vi "Master3.vi"   [LabVIEW 2016, in "Moving Motor.lvrbt"]
uses:
  Moving Motor.lvrbt
  <vilib>/NXT/Block Support/NXT_InputPort.ctl
  <vilib>/NXT/Hardware/Plugins/Tetrix DC Motor/TetrixDCMotorAddress.ctl
  <vilib>/NXT/Hardware/Plugins/Tetrix 180 deg Servo/Tetrix180ServoAddress.ctl
  <vilib>/NXT/Dual Mode Library/Sensors/EV3_Color_Color.vi
  <vilib>/NXT/NXTIO Xnodes/NXTIONodeSubVIs/TETRIX IO Move Servos.vi
  <vilib>/NXT/NXTIO Xnodes/NXTIONodeSubVIs/TETRIX IO Move DC Motors.vi
  <vilib>/NXT/NXTIO Xnodes/NXTIONodeSubVIs/TETRIX IO Stop DC Motors.vi
  <vilib>/NXT/NXTIO Xnodes/AddressXNode/NXTIOAddress.xnode
  <vilib>/NXT/NXTIO Xnodes/NXTIOXNode/NXTIO.xnode
  <vilib>/NXT/Subs/LVHSConnector.ctl
  <vilib>/NXT/LegoClasses/BrickReference/BrickReference.lvclass
types:
  T1 = typedef "NXT_InputPort.ctl" = u32
  T2 = typedef "LVHSConnector.ctl" = refnum<class "BrickReference.lvclass">
  T3 = typedef "Tetrix180ServoAddress.ctl" = i32
  T4 = cluster{"Tetrix180Servo":T3, "Tetrix180Servo":T3}
  T5 = typedef "TetrixDCMotorAddress.ctl" = i32
  T6 = cluster{"TetrixDCMotor":T5, "TetrixDCMotor 2":T5}
  T7 = typedef "ColorSensorColors.ctl" = enum16{"No Color", "Black", "Blue", "Green", "Yellow", "Red", "White", "Brown"}
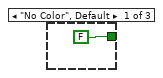
[diagram p2: hidden frame]
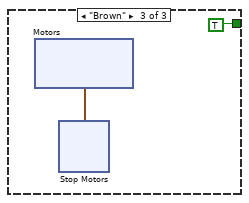
[diagram p3: hidden frame]
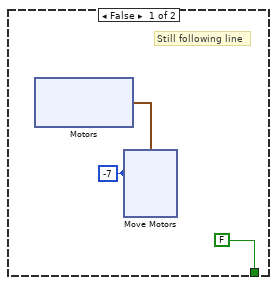
[diagram p4: hidden frame]
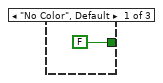
[diagram p5: hidden frame]
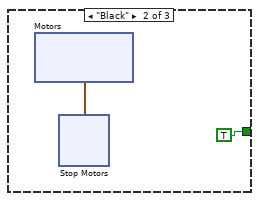
[diagram p6: hidden frame]
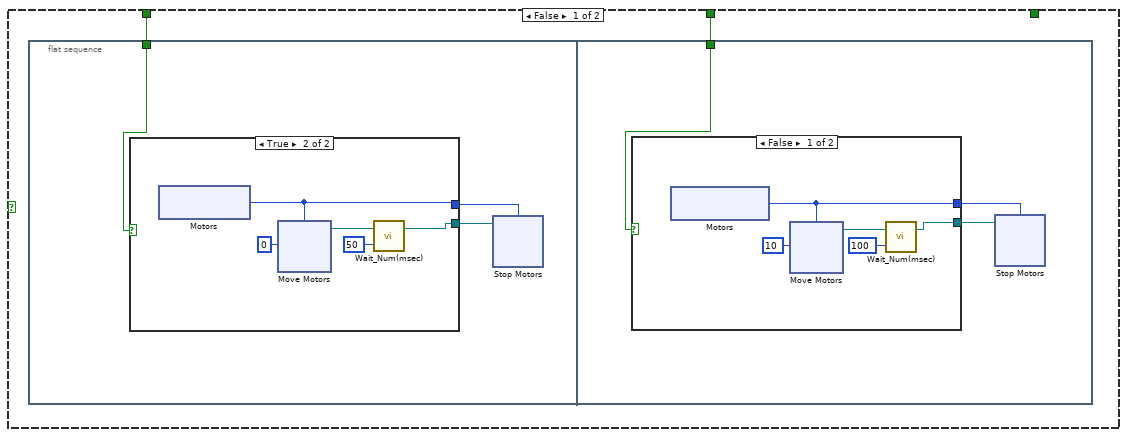
[diagram p7: hidden frame]
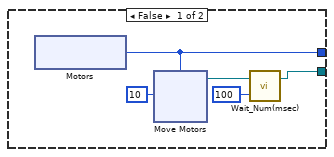
[diagram p8: hidden frame]
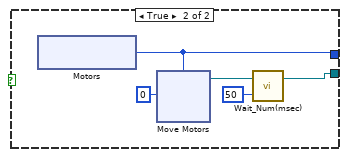
[diagram p9: hidden frame]
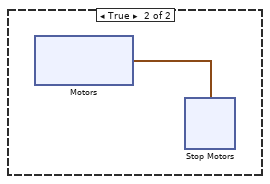
[diagram p10: hidden frame]
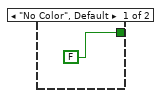
[diagram p11: hidden frame]
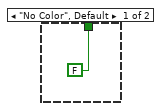
[diagram p12: hidden frame]
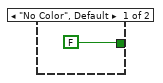
[diagram p13: hidden frame]
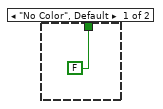
[diagram p14: hidden frame]
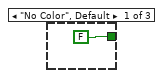
[diagram p15: hidden frame]
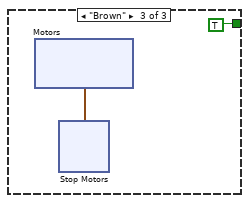
[diagram p16: hidden frame]
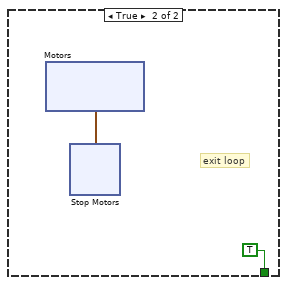
[diagram p17: hidden frame]
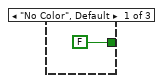
[diagram p18: hidden frame]
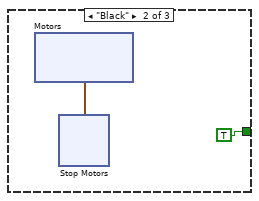
[diagram p19: hidden frame]
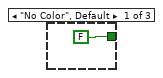
[diagram p20: hidden frame]
diagram:
  w2 = i8 8 ("Power/Speed 1")
  w12 = i8 -16 ("Power/Speed 1")
  w31 = i8 10 ("Power/Speed 1")
  w33 = i8 0 ("Power/Speed 1")
  w45 = i8 -8 ("Power/Speed 1")
  w50 = T1 5 items=["Port 1"=0, "Port 2"=1, "Port 3"=2, "Port 4"=3, "MidRightColor"=5] ("Port (Port 1)")
  w51 = T1 6 items=["Port 1"=0, "Port 2"=1, "Port 3"=2, "Port 4"=3, "MidLeftColor"=6] ("Port (Port 1)")
  w52 = T1 4 items=["Port 1", "Port 2", "Port 3", "Port 4", "RightColor"] ("Port (Port 1)")
  w53 = T1 7 items=["Port 1"=0, "Port 2"=1, "Port 3"=2, "Port 4"=3, "LeftColor"=7] ("Port (Port 1)")
  w70 = i8 -8 ("Power/Speed 1")
  w81 = i8 10 ("Power/Speed 1")
  w80 = i8 0 ("Power/Speed 1")
  # "arm lifting"
  # "Go forward"
  # "Initialize"
  # "Go to intersection"
  # "Turn right"
  # "Combination of line follower and dual-edge detector"
  # "Move backward and turn right to enter the line"
  # "Stop this motor instance"
  # "Stop when it detects the first fat tape"
  # "Let it run for 1s to pass that first thin tape"
  # "Initialize"
  n1 = call-poly <vilib>:"PolySensor.vi"("Port (Port 1)"=w52) -> ("NXT/EV3"=w49:T2)  [unwired: 2 in, 1 out]
  n2 = call-poly <vilib>:"PolySensor.vi"("NXT/EV3"=w49, "Port (Port 1)"=w50) -> ("NXT/EV3"=w48:T2)  [unwired: 1 in, 1 out]
  n3 = call-poly <vilib>:"PolySensor.vi"("NXT/EV3"=w48, "Port (Port 1)"=w51) -> ("NXT/EV3"=w47:T2)  [unwired: 1 in, 1 out]
  n4 = call-poly <vilib>:"PolySensor.vi"("NXT/EV3"=w47, "Port (Port 1)"=w53) -> ("NXT/EV3"=w46:T2)  [unwired: 1 in, 1 out]
  n5 = xnode "Motors"() -> ("Motor"=w78:T4)
  n6 = xnode "Move Servos"("Position 2"=u8 0, "Position 1"=u8 0, "Motors"=w78, "NXT/EV3"=w46) -> ("NXT/EV3"=w79:T2)
  n7 = xnode "Motors"() -> ("Motor"=w58:cluster{"TetrixDCMotor":T5, "TetrixDCMotor":T5})
  n8 = xnode "Move Motors"("Power/Speed 2"=w80, "Power/Speed 1"=w80, "Motors"=w58, "NXT/EV3"=w79) -> ("NXT/EV3"=w86:T2)
  n9 = call <vilib>:"Wait_Num(msec).vi"("Time (100 msec)"=u32 100, "NXT/EV3"=w86) -> ("NXT/EV3"=w82:T2)  [unwired: 2 in]
  n10 = xnode "Move Motors"("Power/Speed 2"=w81, "Power/Speed 1"=w81, "Motors"=w58, "NXT/EV3"=w82) -> ("NXT/EV3"=w84:T2)
  n11 = call <vilib>:"Wait_Num(msec).vi"("Time (100 msec)"=u32 1200, "NXT/EV3"=w84) -> ("NXT/EV3"=w59:T2)  [unwired: 2 in]
  n12 = xnode "Stop Motors"("Motors"=w58, "NXT/EV3"=w59) -> ("NXT/EV3"=w56:T2)
  n13 = call <vilib>:"Wait_Num(msec).vi"("Time (100 msec)"=u32 500, "NXT/EV3"=w56) -> ("NXT/EV3"=w55:T2)  [unwired: 2 in]
  n14 = while {
    tunnel: [w90] -> w72
    tunnel: w55 -> [w87]
    stop <- w91 stop-if-true
    w94 = T1 4 items=["Port 1", "Port 2", "Port 3", "Port 4", "RightColor"] ("Port (Port 1)")
    w96 = T1 7 items=["Port 1"=0, "Port 2"=1, "Port 3"=2, "Port 4"=3, "LeftColor"=7] ("Port (Port 1)")
    n15 = call-poly <vilib>:"PolySensor.vi"("Port (Port 1)"=w96) -> ("Detected Color"=w95:T7)  [unwired: 2 in, 1 out]
    n16 = call-poly <vilib>:"PolySensor.vi"("Port (Port 1)"=w94) -> ("Detected Color"=w93:T7)  [unwired: 2 in, 1 out]
    n17 = case shown="\"Black\"" w95 {
      tunnel: [FALSE TRUE TRUE] -> w89
      tunnel: w87 -> [_ w139 _]
      tunnel: w87 -> [_ _ w148]
      frame "No Color", Default {
      }
      frame "Black" {
        n18 = xnode "Motors"() -> ("Motor"=w141:cluster{"TetrixDCMotor":T5, "TetrixDCMotor":T5})
        n19 = xnode "Stop Motors"("Motors"=w141, "NXT/EV3"=w139) -> ()  [unwired: 1 out]
      }
      frame "Brown" {
        n20 = xnode "Motors"() -> ("Motor"=w149:cluster{"TetrixDCMotor":T5, "TetrixDCMotor":T5})
        n21 = xnode "Stop Motors"("Motors"=w149, "NXT/EV3"=w148) -> ()  [unwired: 1 out]
      }
    }
    n22 = case shown="\"Black\"" w93 {
      tunnel: [FALSE TRUE TRUE] -> w88
      tunnel: w87 -> [_ w98 w107]
      frame "No Color", Default {
      }
      frame "Black" {
        n23 = xnode "Motors"() -> ("Motor"=w99:cluster{"TetrixDCMotor":T5, "TetrixDCMotor":T5})
        n24 = xnode "Stop Motors"("Motors"=w99, "NXT/EV3"=w98) -> ()  [unwired: 1 out]
      }
      frame "Brown" {
        n25 = xnode "Motors"() -> ("Motor"=w108:cluster{"TetrixDCMotor":T5, "TetrixDCMotor":T5})
        n26 = xnode "Stop Motors"("Motors"=w108, "NXT/EV3"=w107) -> ()  [unwired: 1 out]
      }
    }
    n27 = Or(x=w89, y=w88) -> (x .or. y?=w92:bool)
    n28 = case shown="False" w92 {
      tunnel: [FALSE TRUE] -> w91
      tunnel: [w116 w129] -> w90
      frame False {
        w119 = i8 5 ("Power/Speed 1")
        n29 = xnode "Motors"() -> ("Motor"=w118:cluster{"TetrixDCMotor":T5, "TetrixDCMotor":T5})
        n30 = xnode "Move Motors"("Power/Speed 2"=w119, "Power/Speed 1"=w119, "Motors"=w118) -> ("NXT/EV3"=w116:T2)  [unwired: 1 in]
      }
      frame True {
        n31 = xnode "Motors"() -> ("Motor"=w130:cluster{"TetrixDCMotor":T5, "TetrixDCMotor":T5})
        n32 = xnode "Stop Motors"("Motors"=w130) -> ("NXT/EV3"=w129:T2)  [unwired: 1 in]
      }
    }
  }
  n33 = call <vilib>:"Wait_Num(msec).vi"("Time (100 msec)"=u32 1000, "NXT/EV3"=w72) -> ("NXT/EV3"=w71:T2)  [unwired: 2 in]
  n34 = xnode "Motors"() -> ("Motor"=w63:cluster{"TetrixDCMotor":T5, "TetrixDCMotor":T5})
  n35 = xnode "Move Motors"("Power/Speed 2"=w70, "Power/Speed 1"=w70, "Motors"=w63, "NXT/EV3"=w71) -> ("NXT/EV3"=w68:T2)
  n36 = call <vilib>:"Wait_Num(msec).vi"("Time (100 msec)"=u32 700, "NXT/EV3"=w68) -> ("NXT/EV3"=w64:T2)  [unwired: 2 in]
  n37 = xnode "Stop Motors"("Motors"=w63, "NXT/EV3"=w64) -> ("NXT/EV3"=w62:T2)
  n38 = xnode "Move Motors"("Power/Speed 2"=i8 0, "Power/Speed 1"=i8 16, "Motors"=w63, "NXT/EV3"=w62) -> ("NXT/EV3"=w65:T2)
  n39 = call <vilib>:"Wait_Num(msec).vi"("Time (100 msec)"=u32 1800, "NXT/EV3"=w65) -> ("NXT/EV3"=w74:T2)  [unwired: 2 in]
  n40 = xnode "Stop Motors"("Motors"=w63, "NXT/EV3"=w74) -> ("NXT/EV3"=w60:T2)
  n41 = call <vilib>:"Wait_Num(msec).vi"("Time (100 msec)"=u32 1000, "NXT/EV3"=w60) -> ("NXT/EV3"=w54:T2)  [unwired: 2 in]
  n42 = while {
    tunnel: [w157] -> w43
    tunnel: w54 -> [_]
    stop <- w160 stop-if-true
    w163 = T1 7 items=["Port 1"=0, "Port 2"=1, "Port 3"=2, "Port 4"=3, "LeftColor"=4, "RightColor"=7] ("Port (Port 1)")
    w165 = T1 4 items=["Port 1"=0, "Port 2"=1, "Port 3"=2, "Port 4"=3, "LeftColor"=4, "RightColor"=7] ("Port (Port 1)")
    n43 = call-poly <vilib>:"PolySensor.vi"("Port (Port 1)"=w165) -> ("Detected Color"=w164:T7)  [unwired: 2 in, 1 out]
    n44 = call-poly <vilib>:"PolySensor.vi"("Port (Port 1)"=w163) -> ("Detected Color"=w162:T7, "NXT/EV3"=w157:T2)  [unwired: 2 in]
    n45 = case shown="\"Brown\"" w164 {
      tunnel: [FALSE TRUE TRUE] -> w159
      frame "No Color", Default {
      }
      frame "Black" {
        n46 = xnode "Motors"() -> ("Motor"=w205:cluster{"TetrixDCMotor":T5, "TetrixDCMotor":T5})
        n47 = xnode "Stop Motors"("Motors"=w205) -> ()  [unwired: 1 in, 1 out]
      }
      frame "Brown" {
        n48 = xnode "Motors"() -> ("Motor"=w212:cluster{"TetrixDCMotor":T5, "TetrixDCMotor":T5})
        n49 = xnode "Stop Motors"("Motors"=w212) -> ()  [unwired: 1 in, 1 out]
      }
    }
    n50 = case shown="\"Black\"" w162 {
      tunnel: [FALSE TRUE TRUE] -> w158
      frame "No Color", Default {
      }
      frame "Black" {
        n51 = xnode "Motors"() -> ("Motor"=w167:cluster{"TetrixDCMotor":T5, "TetrixDCMotor":T5})
        n52 = xnode "Stop Motors"("Motors"=w167) -> ()  [unwired: 1 in, 1 out]
      }
      frame "Brown" {
        n53 = xnode "Motors"() -> ("Motor"=w175:cluster{"TetrixDCMotor":T5, "TetrixDCMotor":T5})
        n54 = xnode "Stop Motors"("Motors"=w175) -> ()  [unwired: 1 in, 1 out]
      }
    }
    n55 = Or(x=w159, y=w158) -> (x .or. y?=w161:bool)
    n56 = case shown="False" w161 {
      tunnel: [FALSE TRUE] -> w160
      frame False {
        w184 = i8 7 ("Power/Speed 1")
        # "Still following line"
        n57 = xnode "Motors"() -> ("Motor"=w183:cluster{"TetrixDCMotor":T5, "TetrixDCMotor":T5})
        n58 = xnode "Move Motors"("Power/Speed 2"=w184, "Power/Speed 1"=w184, "Motors"=w183) -> ()  [unwired: 1 in, 1 out]
      }
      frame True {
        # "exit loop"
        n59 = xnode "Motors"() -> ("Motor"=w195:cluster{"TetrixDCMotor":T5, "TetrixDCMotor":T5})
        n60 = xnode "Stop Motors"("Motors"=w195) -> ()  [unwired: 1 in, 1 out]
      }
    }
  }
  n61 = call <vilib>:"Wait_Num(msec).vi"("Time (100 msec)"=u32 200, "NXT/EV3"=w43) -> ("NXT/EV3"=w42:T2)  [unwired: 2 in]
  n62 = xnode "Motors"() -> ("Motor"=w44:cluster{"TetrixDCMotor":T5, "TetrixDCMotor":T5})
  n63 = xnode "Move Motors"("Power/Speed 2"=w45, "Power/Speed 1"=w45, "Motors"=w44, "NXT/EV3"=w42) -> ("NXT/EV3"=w39:T2)
  n64 = call <vilib>:"Wait_Num(msec).vi"("Time (100 msec)"=u32 500, "NXT/EV3"=w39) -> ("NXT/EV3"=w38:T2)  [unwired: 2 in]
  n65 = while {
    tunnel: w38 -> [_]
    tunnel: [w220] -> w36
    stop <- w221 stop-if-true
    w232 = T1 5 items=["Port 1"=0, "Port 2"=1, "Port 3"=2, "Port 4"=3, "MidRightColor"=5] ("Port (Port 1)")
    w233 = T1 6 items=["Port 1"=0, "Port 2"=1, "Port 3"=2, "Port 4"=3, "MidLeftColor"=6] ("Port (Port 1)")
    w234 = T1 4 items=["Port 1", "Port 2", "Port 3", "Port 4", "RightColor"] ("Port (Port 1)")
    w235 = T1 7 items=["Port 1"=0, "Port 2"=1, "Port 3"=2, "Port 4"=3, "LeftColor"=7] ("Port (Port 1)")
    n66 = call-poly <vilib>:"PolySensor.vi"("Port (Port 1)"=w234) -> ("Detected Color"=w228:T7, "NXT/EV3"=w220:T2)  [unwired: 2 in]
    n67 = call-poly <vilib>:"PolySensor.vi"("Port (Port 1)"=w235) -> ("Detected Color"=w231:T7)  [unwired: 2 in, 1 out]
    n68 = call-poly <vilib>:"PolySensor.vi"("Port (Port 1)"=w233) -> ("Detected Color"=w230:T7)  [unwired: 2 in, 1 out]
    n69 = call-poly <vilib>:"PolySensor.vi"("Port (Port 1)"=w232) -> ("Detected Color"=w229:T7)  [unwired: 2 in, 1 out]
    n70 = case shown="\"Black\"" w231 {
      tunnel: [FALSE TRUE] -> w224
      frame "No Color", Default {
      }
      frame "Black" {
      }
    }
    n71 = case shown="\"Black\"" w230 {
      tunnel: [FALSE TRUE] -> w227
      frame "No Color", Default {
      }
      frame "Black" {
      }
    }
    n72 = case shown="\"Black\"" w229 {
      tunnel: [FALSE TRUE] -> w226
      frame "No Color", Default {
      }
      frame "Black" {
      }
    }
    n73 = case shown="\"Black\"" w228 {
      tunnel: [FALSE TRUE] -> w223
      frame "No Color", Default {
      }
      frame "Black" {
      }
    }
    n74 = And "LC & RC"(x=w224, y=w223) -> (x .and. y?=w225:bool)
    n75 = And "MLC & MRC"(x=w227, y=w226) -> (x .and. y?=w222:bool)
    n76 = case shown="True" w225 {
      tunnel: w224 -> [w237 _]
      tunnel: w223 -> [w236 _]
      tunnel: w222 -> [_ w306]
      frame False {
        n77 = flat-sequence {
          tunnel: w237 -> [w238]
          tunnel: w236 -> [w272]
          frame #0 {
            n78 = case shown="True" w238 {
              tunnel: [w247 w259] -> w240
              tunnel: [w246 w260] -> w239
              frame False {
                n79 = xnode "Motors"() -> ("Motor"=w246:T5)
                n80 = xnode "Move Motors"("Power/Speed 1"=i8 10, "Motors"=w246) -> ("NXT/EV3"=w249:T2)  [unwired: 1 in]
                n81 = call <vilib>:"Wait_Num(msec).vi"("Time (100 msec)"=u32 100, "NXT/EV3"=w249) -> ("NXT/EV3"=w247:T2)  [unwired: 2 in]
              }
              frame True {
                n82 = xnode "Motors"() -> ("Motor"=w260:T5)
                n83 = xnode "Move Motors"("Power/Speed 1"=i8 0, "Motors"=w260) -> ("NXT/EV3"=w262:T2)  [unwired: 1 in]
                n84 = call <vilib>:"Wait_Num(msec).vi"("Time (100 msec)"=u32 50, "NXT/EV3"=w262) -> ("NXT/EV3"=w259:T2)  [unwired: 2 in]
              }
            }
            n85 = xnode "Stop Motors"("Motors"=w239, "NXT/EV3"=w240) -> ()  [unwired: 1 out]
          }
          frame #1 {
            n86 = case shown="False" w272 {
              tunnel: [w281 w293] -> w274
              tunnel: [w280 w294] -> w273
              frame False {
                n87 = xnode "Motors"() -> ("Motor"=w280:T5)
                n88 = xnode "Move Motors"("Power/Speed 1"=i8 10, "Motors"=w280) -> ("NXT/EV3"=w283:T2)  [unwired: 1 in]
                n89 = call <vilib>:"Wait_Num(msec).vi"("Time (100 msec)"=u32 100, "NXT/EV3"=w283) -> ("NXT/EV3"=w281:T2)  [unwired: 2 in]
              }
              frame True {
                n90 = xnode "Motors"() -> ("Motor"=w294:T5)
                n91 = xnode "Move Motors"("Power/Speed 1"=i8 0, "Motors"=w294) -> ("NXT/EV3"=w296:T2)  [unwired: 1 in]
                n92 = call <vilib>:"Wait_Num(msec).vi"("Time (100 msec)"=u32 50, "NXT/EV3"=w296) -> ("NXT/EV3"=w293:T2)  [unwired: 2 in]
              }
            }
            n93 = xnode "Stop Motors"("Motors"=w273, "NXT/EV3"=w274) -> ()  [unwired: 1 out]
          }
        }
      }
      frame True {
        n94 = case shown="False" w306 {
          frame False {
            n95 = xnode "Motors"() -> ("Motor"=w312:cluster{"TetrixDCMotor":T5, "TetrixDCMotor":T5})
            n96 = xnode "Stop Motors"("Motors"=w312) -> ("NXT/EV3"=w318:T2)  [unwired: 1 in]
            n97 = call <vilib>:"Wait_Num(msec).vi"("Time (100 msec)"=u32 50, "NXT/EV3"=w318) -> ("NXT/EV3"=w313:T2)  [unwired: 2 in]
            n98 = xnode "Move Motors"("Power/Speed 2"=i8 0, "Power/Speed 1"=i8 -9, "Motors"=w312, "NXT/EV3"=w313) -> ("NXT/EV3"=w315:T2)
            n99 = call <vilib>:"Wait_Num(msec).vi"("Time (100 msec)"=u32 800, "NXT/EV3"=w315) -> ("NXT/EV3"=w319:T2)  [unwired: 2 in]
            n100 = xnode "Stop Motors"("Motors"=w312, "NXT/EV3"=w319) -> ("NXT/EV3"=w309:T2)
            n101 = xnode "Move Motors"("Power/Speed 2"=i8 -9, "Power/Speed 1"=i8 0, "Motors"=w312, "NXT/EV3"=w309) -> ("NXT/EV3"=w307:T2)
            n102 = call <vilib>:"Wait_Num(msec).vi"("Time (100 msec)"=u32 800, "NXT/EV3"=w307) -> ()  [unwired: 2 in, 1 out]
          }
          frame True {
            n103 = xnode "Motors"() -> ("Motor"=w348:cluster{"TetrixDCMotor":T5, "TetrixDCMotor":T5})
            n104 = xnode "Stop Motors"("Motors"=w348) -> ()  [unwired: 1 in, 1 out]
          }
        }
      }
    }
    n105 = And "Only exit loop when all 4 sensors detect black"(x=w225, y=w222) -> (x .and. y?=w221:bool)
  }
  n106 = xnode "Motors"() -> ("Motor"=w17:T4)
  n107 = call <vilib>:"Wait_Num(msec).vi"("Time (100 msec)"=u32 200, "NXT/EV3"=w36) -> ("NXT/EV3"=w19:T2)  [unwired: 2 in]
  n108 = xnode "Move Servos"("Position 2"=u8 54, "Position 1"=u8 0, "Motors"=w17, "NXT/EV3"=w19) -> ("NXT/EV3"=w32:T2)
  n109 = xnode "Motors"() -> ("Motor"=w24:cluster{"TetrixDCMotor":T5, "TetrixDCMotor":T5})
  n110 = xnode "Move Motors"("Power/Speed 2"=w33, "Power/Speed 1"=w33, "Motors"=w24, "NXT/EV3"=w32) -> ("NXT/EV3"=w28:T2)
  n111 = xnode "Move Motors"("Power/Speed 2"=w31, "Power/Speed 1"=w31, "Motors"=w24, "NXT/EV3"=w28) -> ("NXT/EV3"=w29:T2)
  n112 = call-poly <vilib>:"PolyWait.vi"("Time (100 msec)"=u32 1000, "NXT/EV3"=w29) -> ("NXT/EV3"=w27:T2)  [unwired: 2 in]
  n113 = xnode "Stop Motors"("Motors"=w24, "NXT/EV3"=w27) -> ("NXT/EV3"=w22:T2)
  n114 = xnode "Move Servos"("Position 2"=u8 0, "Position 1"=u8 0, "Motors"=w17, "NXT/EV3"=w22) -> ("NXT/EV3"=w20:T2)
  n115 = call-poly <vilib>:"PolyWait.vi"("Time (100 msec)"=u32 2000, "NXT/EV3"=w20) -> ("NXT/EV3"=w15:T2)  [unwired: 2 in]
  n116 = xnode "Move Servos"("Position 2"=u8 120, "Position 1"=u8 100, "Motors"=w17, "NXT/EV3"=w15) -> ("NXT/EV3"=w14:T2)
  n117 = call-poly <vilib>:"PolyWait.vi"("Time (100 msec)"=u32 4000, "NXT/EV3"=w14) -> ("NXT/EV3"=w13:T2)  [unwired: 2 in]
  n118 = while {
    tunnel: [w363] -> w3
    tunnel: w13 -> [_]
    stop <- w366 stop-if-true
    w369 = T1 7 items=["Port 1"=0, "Port 2"=1, "Port 3"=2, "Port 4"=3, "LeftColor"=4, "RightColor"=7] ("Port (Port 1)")
    w371 = T1 4 items=["Port 1"=0, "Port 2"=1, "Port 3"=2, "Port 4"=3, "LeftColor"=4, "RightColor"=7] ("Port (Port 1)")
    n119 = call-poly <vilib>:"PolySensor.vi"("Port (Port 1)"=w371) -> ("Detected Color"=w370:T7)  [unwired: 2 in, 1 out]
    n120 = call-poly <vilib>:"PolySensor.vi"("Port (Port 1)"=w369) -> ("Detected Color"=w368:T7, "NXT/EV3"=w363:T2)  [unwired: 2 in]
    n121 = case shown="\"Brown\"" w370 {
      tunnel: [FALSE TRUE TRUE] -> w365
      frame "No Color", Default {
      }
      frame "Black" {
        n122 = xnode "Motors"() -> ("Motor"=w404:cluster{"TetrixDCMotor":T5, "TetrixDCMotor":T5})
        n123 = xnode "Stop Motors"("Motors"=w404) -> ()  [unwired: 1 in, 1 out]
      }
      frame "Brown" {
        n124 = xnode "Motors"() -> ("Motor"=w411:cluster{"TetrixDCMotor":T5, "TetrixDCMotor":T5})
        n125 = xnode "Stop Motors"("Motors"=w411) -> ()  [unwired: 1 in, 1 out]
      }
    }
    n126 = case shown="\"Black\"" w368 {
      tunnel: [FALSE TRUE TRUE] -> w364
      frame "No Color", Default {
      }
      frame "Black" {
        n127 = xnode "Motors"() -> ("Motor"=w373:cluster{"TetrixDCMotor":T5, "TetrixDCMotor":T5})
        n128 = xnode "Stop Motors"("Motors"=w373) -> ()  [unwired: 1 in, 1 out]
      }
      frame "Brown" {
        n129 = xnode "Motors"() -> ("Motor"=w381:cluster{"TetrixDCMotor":T5, "TetrixDCMotor":T5})
        n130 = xnode "Stop Motors"("Motors"=w381) -> ()  [unwired: 1 in, 1 out]
      }
    }
    n131 = Or(x=w365, y=w364) -> (x .or. y?=w367:bool)
    n132 = case shown="True" w367 {
      tunnel: [FALSE TRUE] -> w366
      frame False {
        w390 = i8 -7 ("Power/Speed 1")
        # "Still following line"
        n133 = xnode "Motors"() -> ("Motor"=w389:cluster{"TetrixDCMotor":T5, "TetrixDCMotor":T5})
        n134 = xnode "Move Motors"("Power/Speed 2"=w390, "Power/Speed 1"=w390, "Motors"=w389) -> ()  [unwired: 1 in, 1 out]
      }
      frame True {
        # "exit loop"
      }
    }
  }
  n135 = xnode "Motors"() -> ("Motor"=w4:cluster{"TetrixDCMotor":T5, "TetrixDCMotor":T5})
  n136 = xnode "Move Motors"("Power/Speed 2"=w2, "Power/Speed 1"=w2, "Motors"=w4, "NXT/EV3"=w3) -> ("NXT/EV3"=w5:T2)
  n137 = call <vilib>:"Wait_Num(msec).vi"("Time (100 msec)"=u32 610, "NXT/EV3"=w5) -> ("NXT/EV3"=w1:T2)  [unwired: 2 in]
  n138 = xnode "Motors"() -> ("Motor"=w7:cluster{"TetrixDCMotor":T5, "TetrixDCMotor":T5})
  n139 = Negate(x=w12) -> (-x=w11:i8)
  n140 = xnode "Move Motors"("Power/Speed 2"=w11, "Power/Speed 1"=w12, "Motors"=w7, "NXT/EV3"=w1) -> ("NXT/EV3"=w9:T2)
  n141 = call <vilib>:"Wait_Num(msec).vi"("Time (100 msec)"=u32 1050, "NXT/EV3"=w9) -> ("NXT/EV3"=w8:T2)  [unwired: 2 in]
  n142 = xnode "Stop Motors"("Motors"=w7, "NXT/EV3"=w8) -> ()  [unwired: 1 out]
